vi "Init Measurement Message.vi"(5 "Meaurement Message":refnum<class "TestManagerMsg.Measurement.lvclass">, 7 "overwrite?":bool=TRUE, 8 "Value":variant, 9 "name":string, 10 "self-id":string, 11 "owner-id":string) -> (3 "Message":refnum<class "TestManagerMsg.lvclass">)   [LabVIEW 2013, in "Caraya.lvlib" / "TestManagerMsg.Measurement.lvclass"]
uses:
  TestManagerMsg.Measurement.lvclass
  Test Manager Message/TestManagerMsg.lvclass
  TestManagerMsg.Measurement.lvclass/TestManagerMsg.Measurement.ctl
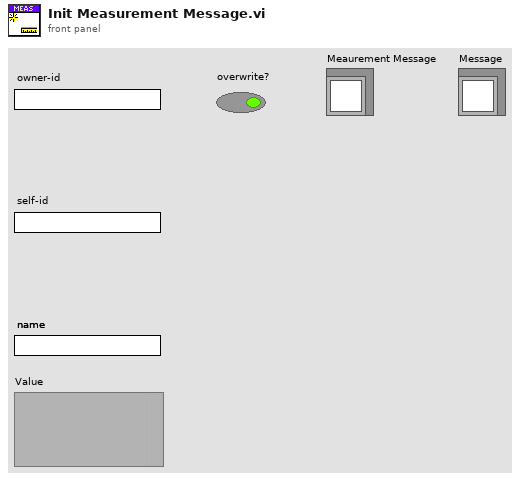
[diagram p1: front panel]
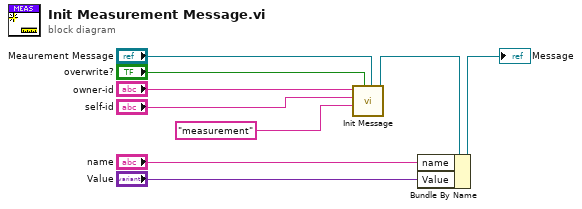
[diagram p0: block diagram]
diagram:
  n1 = call "Init Message.vi"("TestManagerMsg"="Meaurement Message", "overwrite?"="overwrite?", "key"="measurement", "self-id"="self-id", "owner-id"="owner-id") -> ("Message"=w7:refnum<class "TestManagerMsg.Measurement.lvclass">)  [unwired: 6 in]
  n2 = Bundle By Name(cluster=w7, "name"="name", "Value"="Value") -> (→"Message":refnum<class "TestManagerMsg.Measurement.lvclass">)
